vi "Configure Partial Modulation Pause Power.vi"(8 "error in (no error)":errorcluster, 10 "Ppause, W":u16=50, 11 "HFP Gen in":refnum<class "PL HFP Generator.lvclass">) -> (0 "error out":errorcluster, 3 "HFP Gen out":refnum<class "PL HFP Generator.lvclass">)   [LabVIEW 2015, in "PL HFP Generator.lvclass"]
doc: "Configures partial modulation pause power (for Plasma G20 series)."
uses:
  PL HFP Generator.lvclass
  PL HFP Generator.lvclass/PL HFP Generator.ctl
  <vilib>/plasmapper/PL Modbus Client/PL Modbus Client.lvclass
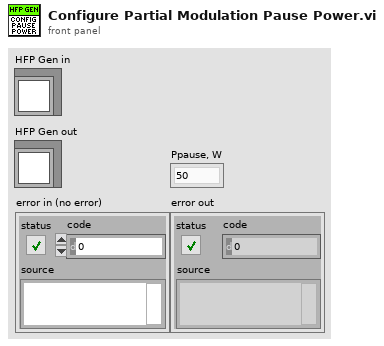
[diagram p1: front panel]
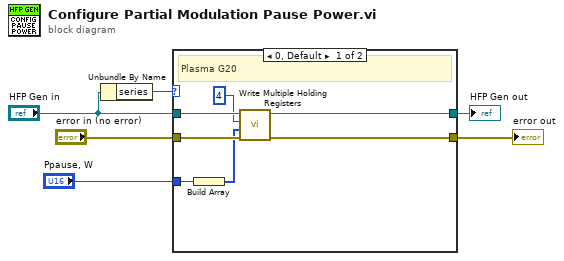
[diagram p0: block diagram]
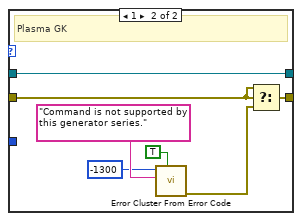
[diagram p2: hidden frame]
diagram:
  n1 = Unbundle By Name("HFP Gen in") -> ("series"=w6:u16)
  n2 = case shown="0, Default" w6 {
    tunnel: [w13 w20] -> w2
    tunnel: [w12 w18] -> w1
    tunnel: "error in (no error)" -> [w11 w19]
    tunnel: "HFP Gen in" -> [w10 w20]
    tunnel: "Ppause, W" -> [w7 _]
    frame 0, Default {
      # "Plasma G20"
      n3 = Build Array(w7) -> (w8:u16[])
      n4 = call <vilib>:"Write Multiple Holding Registers.vi"("error in (no error)"=w11, "values"=w8, "address"=u16 4, "MODBUS in"=w10) -> ("error out"=w12:errorcluster, "MODBUS out"=w13:refnum<class "PL HFP Generator.lvclass">)  [unwired: 6 in]
    }
    frame 1 {
      # "Plasma GK"
      n5 = call <vilib>:"Error Cluster From Error Code.vi"("show call chain? (False)"=TRUE, "error message (\"\")"="Command is not supported by this generator series." ("format string"), "error code (0)"=-1300) -> ("error out"=w14:errorcluster)  [unwired: 6 in]
      n6 = Select(t=w19, s=w19, f=w14) -> (s? t:f=w18:errorcluster)
    }
  }
  "HFP Gen out" <- w2
  "error out" <- w1
